vi "testFluorescenceAnalysis.vi"() -> ()   [LabVIEW 2011, in "run.lvlib"]
uses:
  run.lvlib
  Tools/ImageProcessor/ImageAnalyser/FluorescenceLiveAnalyser/FluorescenceLiveAnalyser.lvclass
panel:
  out "Image":T1(plugin-control)
  in  "stop":bool=TRUE
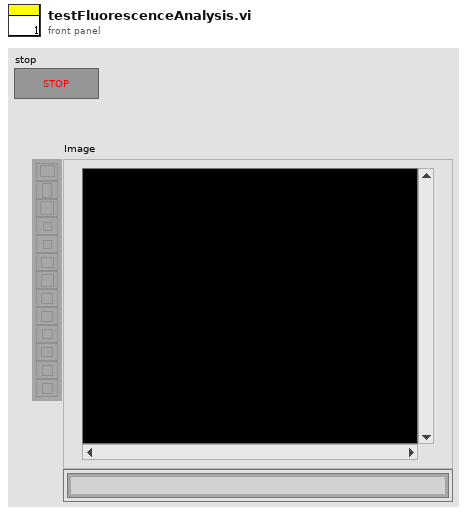
[diagram p1: front panel]
types:
  T1 = typedef "IMAQ Image.ctl" = refnum<image>
  T2 = typedef "Image Type" = u32
  T3 = cluster{"ImageName":string, "ImageArray":sgl[][]}
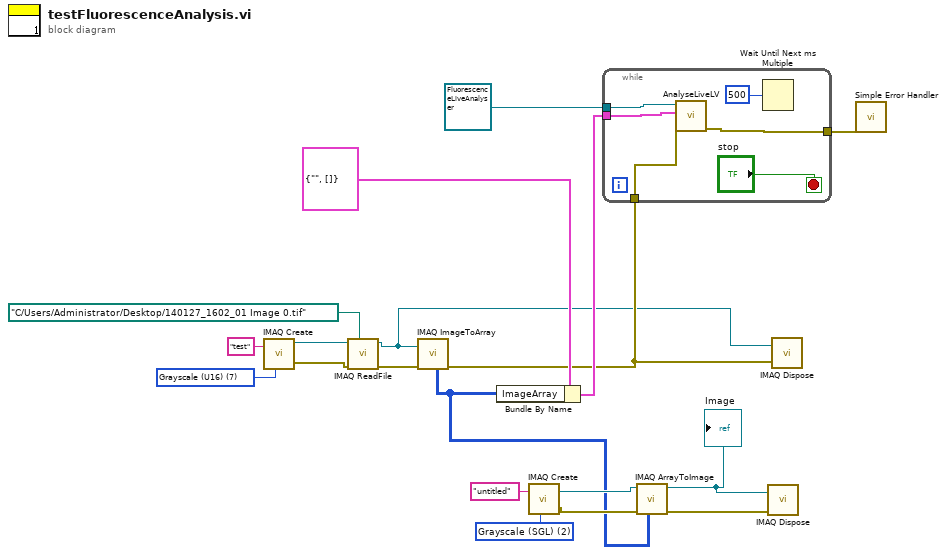
[diagram p0: block diagram]
diagram:
  w6 = T2 2 items=["Grayscale (U8)", "Grayscale (I16)", "Grayscale (SGL)", "Complex (CSG)", "RGB (U32)", "HSL (U32)", "RGB (U64)", "Grayscale (U16)"] ("Image Type")
  w14 = T2 7 items=["Grayscale (U8)", "Grayscale (I16)", "Grayscale (SGL)", "Complex (CSG)", "RGB (U32)", "HSL (U32)", "RGB (U64)", "Grayscale (U16)"] ("Image Type")
  n1 = call "IMAQ Create"("Image Name"="test", "Image Type"=w14) -> ("New Image"=w18:T1, "error out"=w17:errorcluster)  [unwired: 3 in]
  n2 = call "IMAQ ReadFile"("File Path"=path "C:/Users/Administrator/Desktop/140127_1602_01 Image 0.tif", "error in (no error)"=w17, "Image"=w18) -> ("error out"=w15:errorcluster, "Image Out"=w2:T1)  [unwired: 4 in, 3 out]
  n3 = call "IMAQ ImageToArray"("error in (no error)"=w15, "Image"=w2) -> ("Image Pixels (U16)"=w1:u16[][], "error out"=w3:errorcluster)  [unwired: 2 in, 3 out]
  n4 = Bundle By Name(cluster=T3 {"ImageName"="", "ImageArray"=[]} ("ImageData"), "ImageArray"=w1) -> (w11:T3)
  n5 = call "IMAQ Create"("Image Name"="untitled", "Image Type"=w6) -> ("New Image"=w9:T1, "error out"=w8:errorcluster)  [unwired: 3 in]
  n6 = while {
    tunnel: refnum<class "FluorescenceLiveAnalyser.lvclass"> refnum ("FluorescenceLiveAnalyser in") -> [w23]
    tunnel: w11 -> [w22]
    tunnel: w3 -> [w21]
    tunnel: [w20] -> w10
    stop <- "stop" stop-if-true
    n7 = call "AnalyseLiveLV.vi"("error in (no error)"=w21, "ImageData"=w22, "FluorescenceLiveAnalyser in"=w23) -> ("error out"=w20:errorcluster)  [unwired: 7 in, 1 out]
    n8 = Wait Until Next ms Multiple(millisecond multiple=500) -> ()  [unwired: 1 out]
  }
  n9 = call "IMAQ ArrayToImage"("Image Pixels (Float)"=w1, "error in (no error)"=w8, "Image"=w9) -> ("error out"=w5:errorcluster, "Image Out"=w4:T1)  [unwired: 7 in]
  "Image" <- w4
  n10 = call "IMAQ Dispose"("Image"=w4, "error in (no error)"=w5) -> ()  [unwired: 4 in, 1 out]
  n11 = call "IMAQ Dispose"("Image"=w2, "error in (no error)"=w3) -> ()  [unwired: 4 in, 1 out]
  n12 = call <vilib>:"Simple Error Handler.vi"("error in (no error)"=w10) -> ()  [unwired: 4 in, 5 out]
